vi "Main On Compile Action VI Wrapper.vi"(8 "error in (no error)":errorcluster, 11 "Device Item Ref in":T1 format="%.0x") -> (0 "error out":errorcluster)   [LabVIEW 2015, in "Engine Simulation Toolkit System Explorer.lvlib"]
uses:
  Engine Simulation Toolkit System Explorer.lvlib
  <vilib>/NI Veristand/Custom Device API/Custom Device Item Ref.ctl
  Shared/Constants and GUIDs.vi
  Shared/Engine Simulation Toolkit Shared.lvlib
  <vilib>/NI Veristand/Custom Device API/Custom Device API.lvlib
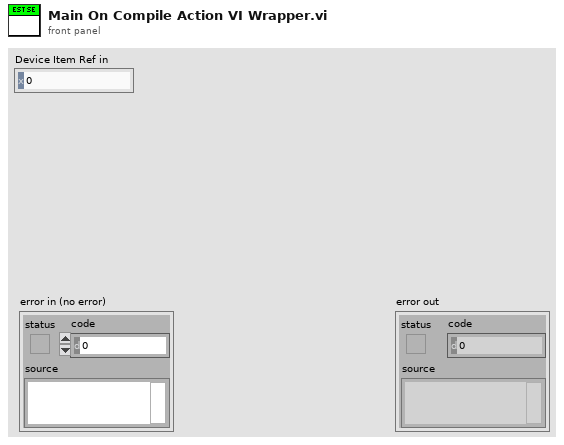
[diagram p1: front panel]
types:
  T1 = typedef "Custom Device API.lvlib/Custom Device Item Ref.ctl" = u64
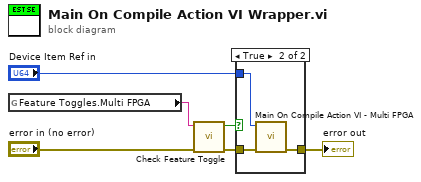
[diagram p0: block diagram]
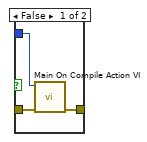
[diagram p2: hidden frame]
diagram:
  n1 = global read "Constants and GUIDs.vi" "Feature Toggles.Multi FPGA"() -> (w6:string)
  n2 = call "Check Feature Toggle.vi"("error in (no error)"="error in (no error)", "feature name"=w6) -> ("error out"=w2:errorcluster, "feature enabled"=w5:bool)  [unwired: 8 in]
  n3 = case shown="True" w5 {
    tunnel: "Device Item Ref in" -> [w7 w12]
    tunnel: w2 -> [w8 w11]
    tunnel: [w9 w10] -> w1
    frame False {
      n4 = call "Main On Compile Action VI.vi"("error in (no error)"=w8, "Device Item Ref in"=w7) -> ("error out"=w9:errorcluster)  [unwired: 9 in]
    }
    frame True {
      n5 = call "Main On Compile Action VI - Multi FPGA.vi"("error in (no error)"=w11, "Device Item Ref in"=w12) -> ("error out"=w10:errorcluster)  [unwired: 9 in]
    }
  }
  "error out" <- w1
